vi "tcp client listen.vi"(8 "error in (no error)":errorcluster, 9 "write Server stats timeout":i32=5000, 11 "listener ID in":refnum<k5>) -> (0 "listen loop error out":errorcluster, 1 "listen halted":bool, 2 "Server Stats out":T1={"scan rate"=10.0, "# connections"=0, "channel settings"=[]} {"channel settings"."lower input limits" format="%.4f"; "channel settings"."upper input limits" format="%.4f"; "scan rate" format="%.2f"})   [LabVIEW 2012]
uses:
  DataServer/Server stats.ctl
panel:
  # "Hz"
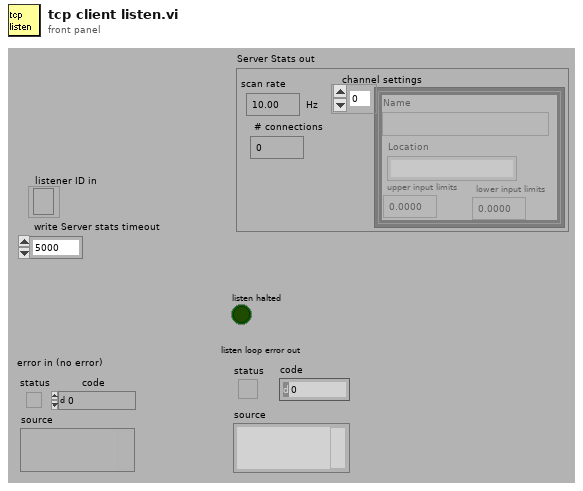
[diagram p1: front panel]
types:
  T1 = typedef "Server stats.ctl" = cluster{"scan rate":dbl, "# connections":i32, "channel settings":cluster{"Name":string, "upper input limits":sgl, "lower input limits":sgl, "Location":string}[]}
  T2 = enum16{"clear", "add connection", "change command", "write state", "delete connection", "read"}
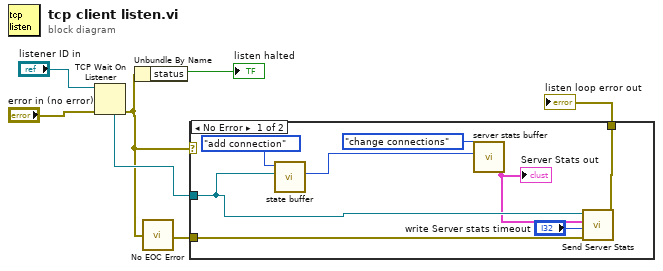
[diagram p0: block diagram]
diagram:
  n1 = TCP Wait On Listener(8:"error in (no error)", 11:"listener ID in") -> (0:w2:errorcluster, 4:w6:refnum<k5>)  [unwired: 2 in, 3 out]
  n2 = Unbundle By Name(w2) -> ("status"=→"listen halted":bool)
  n3 = call "No EOC Error.vi"("error in"=w2) -> ("error out"=w5:errorcluster)  [unwired: 4 in]
  n4 = case shown="No Error" w2 {
    tunnel: w6 -> [w12 _]
    tunnel: w5 -> [w15 w16]
    tunnel: [w14 w16] -> w4
    frame No Error {
      n5 = call "state buffer.vi"("connection"=w12, "command"=T2."add connection") -> ("clients"=w9:i32)  [unwired: 7 in, 2 out]
      n6 = call "server stats buffer.vi"("# connections"=w9, "state"=enum16{"write", "read", "change connections"}."change connections") -> ("Server Stats out"=w8:T1)  [unwired: 5 in]
      "Server Stats out" <- w8
      n7 = call "Send Server Stats.vi"("error in (no error)"=w15, "timeout ms (25000)"="write Server stats timeout", "Server Stats"=w8, "refnum in"=w12) -> ("error out"=w14:errorcluster)  [unwired: 5 in, 2 out]
    }
    frame Error {
    }
  }
  "listen loop error out" <- w4
